vi "pH电极校准.vi"() -> ()   [LabVIEW 2016, in "斯坦道多参数.lvlib"]
uses:
  <vilib>/Utility/miscctls.llb/LVPointTypeDef.ctl
  <vilib>/Analysis/NI_AALBase.lvlib
  <vilib>/ptbypt/NI_PtbyPt.lvlib
panel:
  in  "刷新按钮":bool
  out "第三点信号值":dbl
  out "第二点信号值":dbl
  out "第一点信号值":dbl
  out "温度":dbl format="%#.2f"
  out "通讯状态":string
  out "电极状态标志":u16(ring) items=["OK", "第一点校正通过", "第二点校正通过", "校正失败,电极零点超出范围", "校正失败,电极斜率超出范围", "第三点校正通过"]
  in  "三点标液3":u16(ring)=6 caption="标液3" items=["TECH4.00", "TECH7.00", "TECH10.00", "NIST1.68", "NIST4.01", "NIST6.86", "NIST9.18", "NIST12.68"]
  in  "三点标液2":u16(ring)=5 caption="标液2" items=["TECH4.00", "TECH7.00", "TECH10.00", "NIST1.68", "NIST4.01", "NIST6.86", "NIST9.18", "NIST12.68"]
  in  "三点标液1":u16(ring)=4 caption="标液1" items=["TECH4.00", "TECH7.00", "TECH10.00", "NIST1.68", "NIST4.01", "NIST6.86", "NIST9.18", "NIST12.68"]
  out "第三点校准值":dbl
  in  "校准停止":bool
  in  "校准启动":bool
  out "第二点校准值":dbl
  out "第一点校准值":dbl
  out "提示":string
  in  "校准模式":enum16{"两点校准", "单点校准", "三点校准"}(ring)
  out "最小值":sgl format="%#.2f"
  out "最大值":sgl format="%#.2f"
  out "变异系数":dbl format="%#.6f"
  out "standard deviation":dbl caption="标准差" format="%#.2f"
  out "mean":dbl caption="均值" format="%#.2f"
  out "波形图表":dbl(graph) caption="历史曲线"
  out "当前检测值":dbl caption="测量值" format="%#.2f"
  out "标液2":dbl
  out "标液1":dbl
  out "当前信号值":dbl caption="信号值" format="%#.2f"
  out "偏移值补偿":dbl caption="pH偏移修正值" format="%#.2f"
  out "电极斜率":dbl format="%#.6f"
  out "电极零点":dbl format="%#.6f"
  # "酸碱度电极设定"
  # "℃"
  # "mV"
  # "mV"
  # "%"
  # "请选择校准模式:"
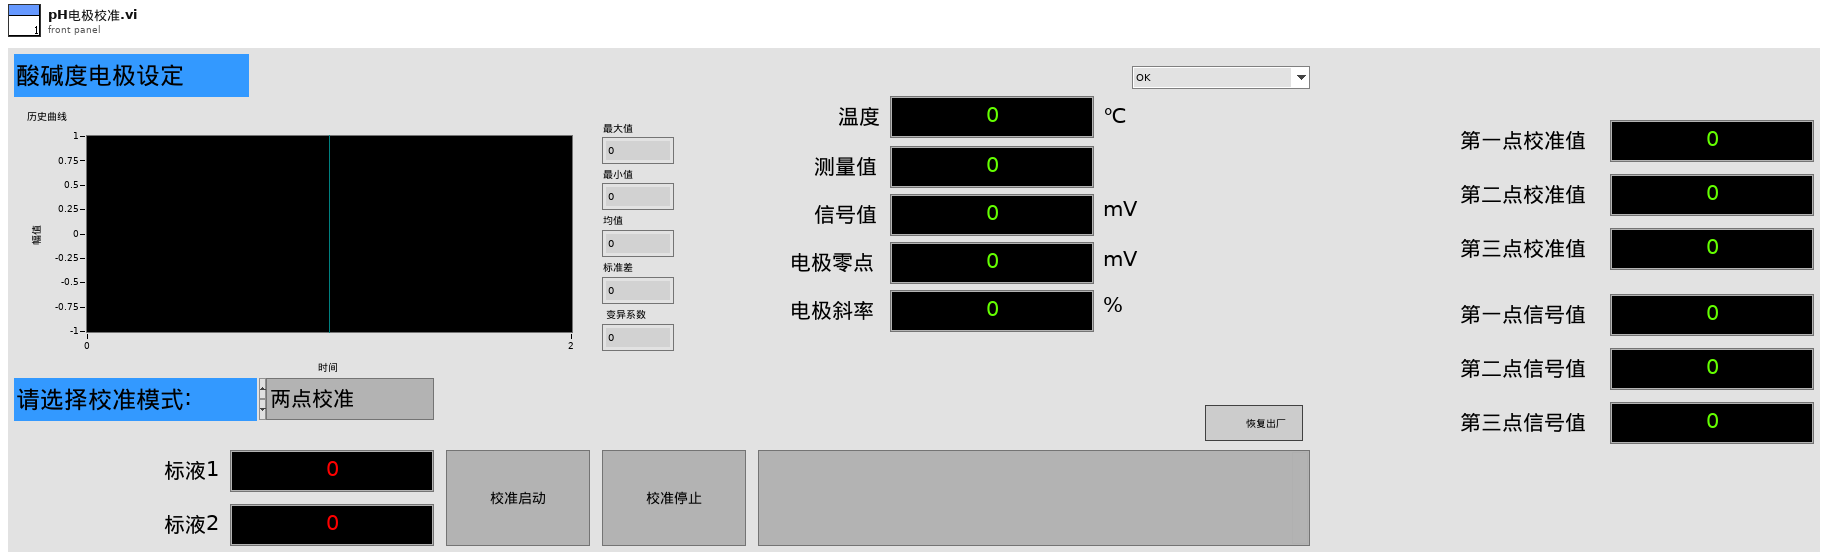
[diagram p1: front panel]
types:
  T1 = typedef "LVPointTypeDef.ctl" = cluster{"Horizontal":i16, "Vertical":i16}
  T2 = cluster{"电极状态标志":u16, "电极型号标志":u16, "酸碱度测量值":sgl, "温度测量值":sgl, "酸碱度信号值":sgl, "温度信号值":sgl, "酸碱度偏移修正值":sgl, "温度偏移修正值":sgl, "手动温度补偿值":sgl, "酸碱度电极零点":sgl, "酸碱度电极斜率":sgl, "第1点标准值记录":sgl, "第1点信号值记录":sgl, "第1点温度值记录":sgl, "第2点标准值记录":sgl, "第2点信号值记录":sgl, "第2点温度值记录":sgl, "命令滤波设定":u16, "温度模式":enum16{"ATC", "MTC"}, "生产批次":u16, "电极序号":u16, "串口地址":u16, "串口波特率":enum16{"9600", "19200", "115200"}, "串口校验位":enum16{"NONE", "ODD", "EVEN"}, "串口停止位":enum16{"1bit", "2bit"}, "第一点标准值":sgl, "第二点标准值":sgl}
  T3 = enum8{"Enabled", "Disabled", "Disabled and Grayed Out"}
  T4 = cluster{"ph":bool, "DO":bool, "Cond":bool, "Turb":bool, "叶绿素a":bool, "藻密度":bool, "ORP":bool}
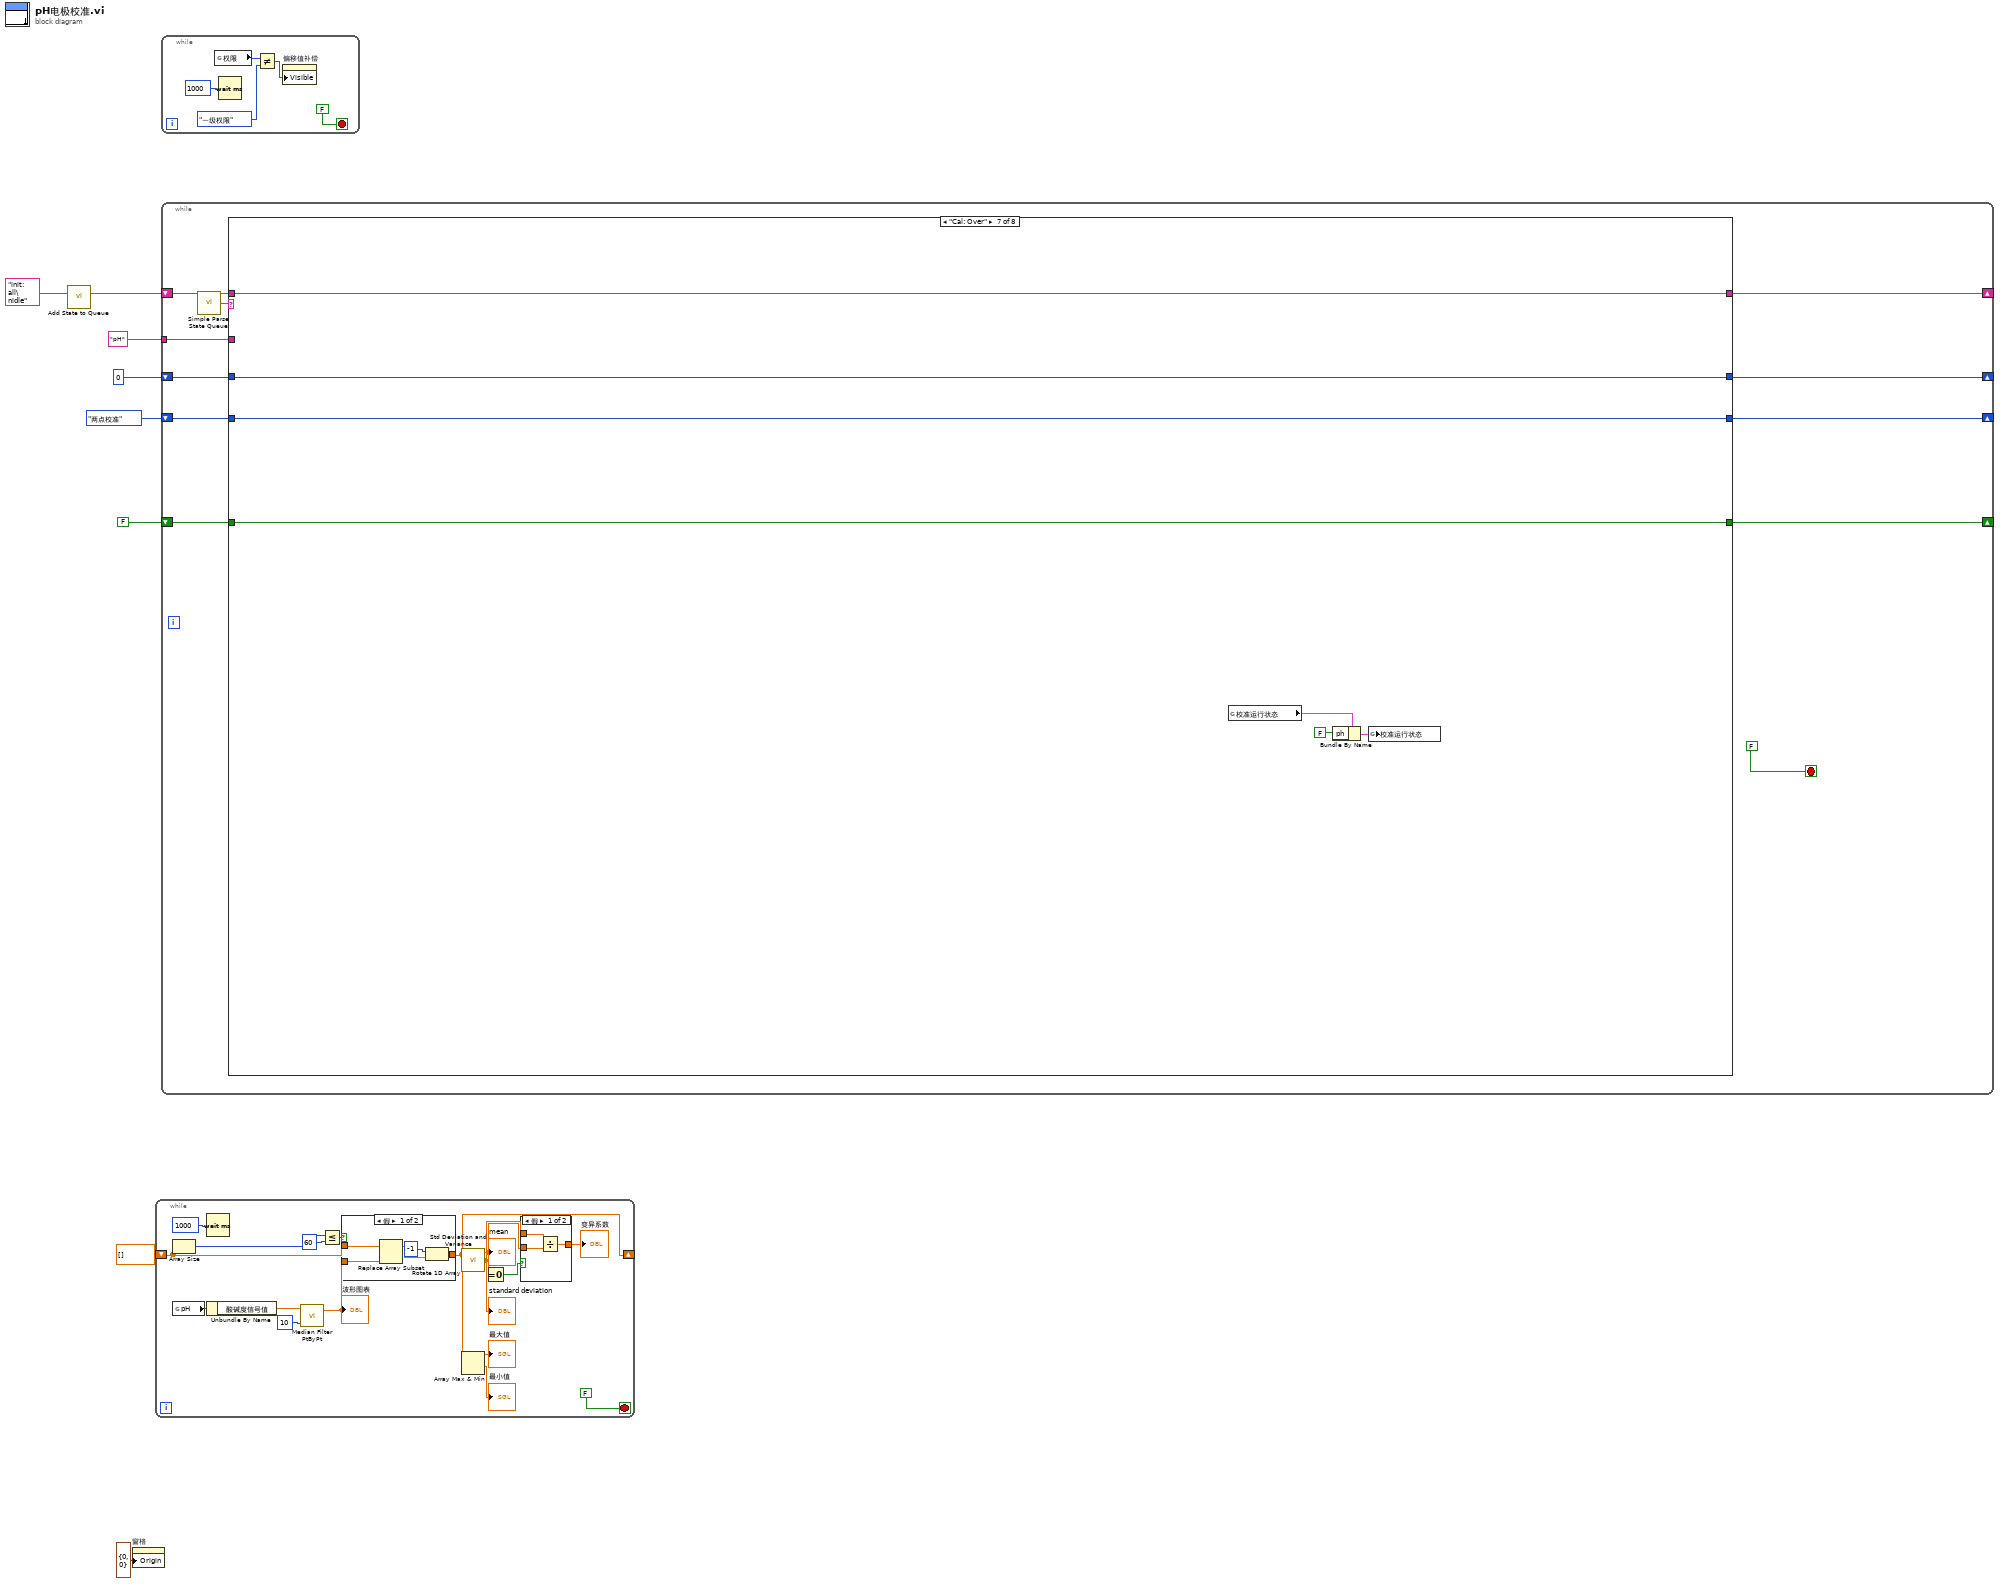
[diagram p0: block diagram]
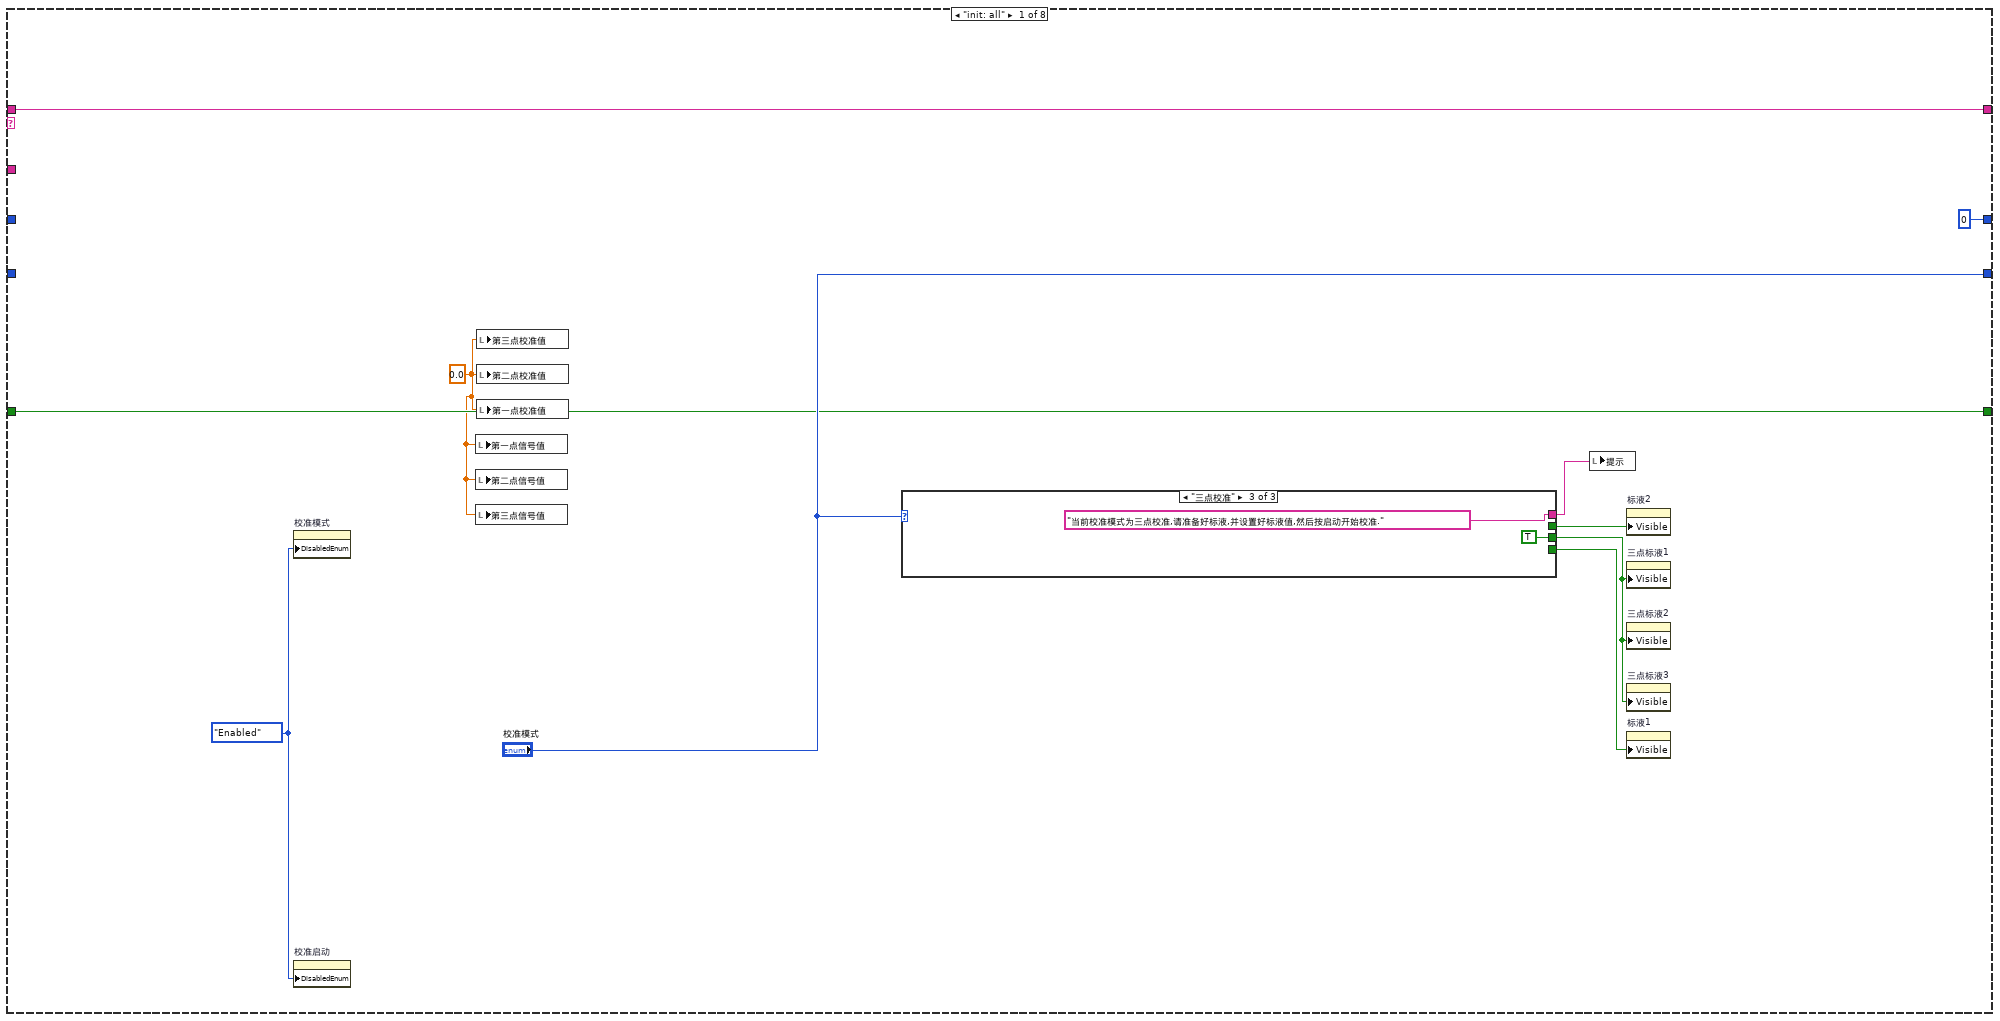
[diagram p2: hidden frame]
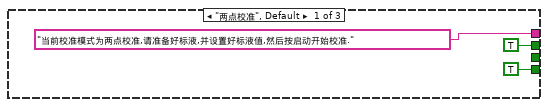
[diagram p3: hidden frame]
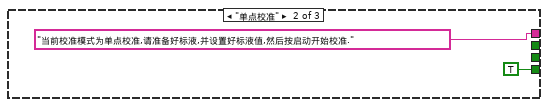
[diagram p4: hidden frame]
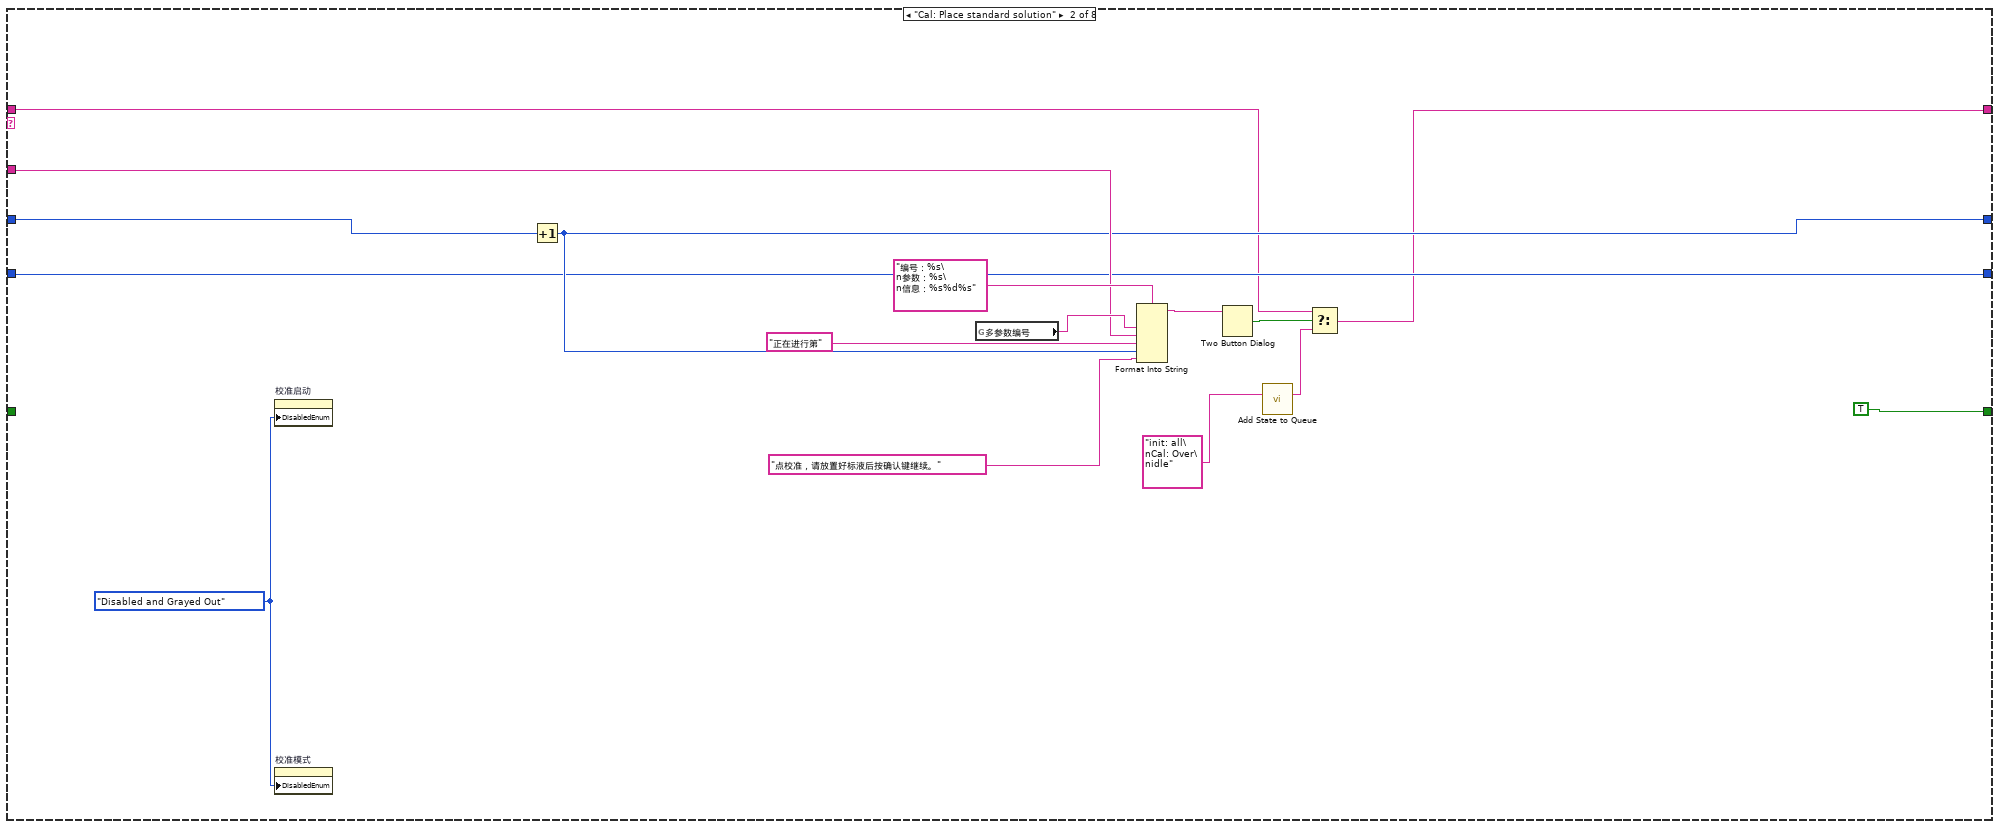
[diagram p5: hidden frame]
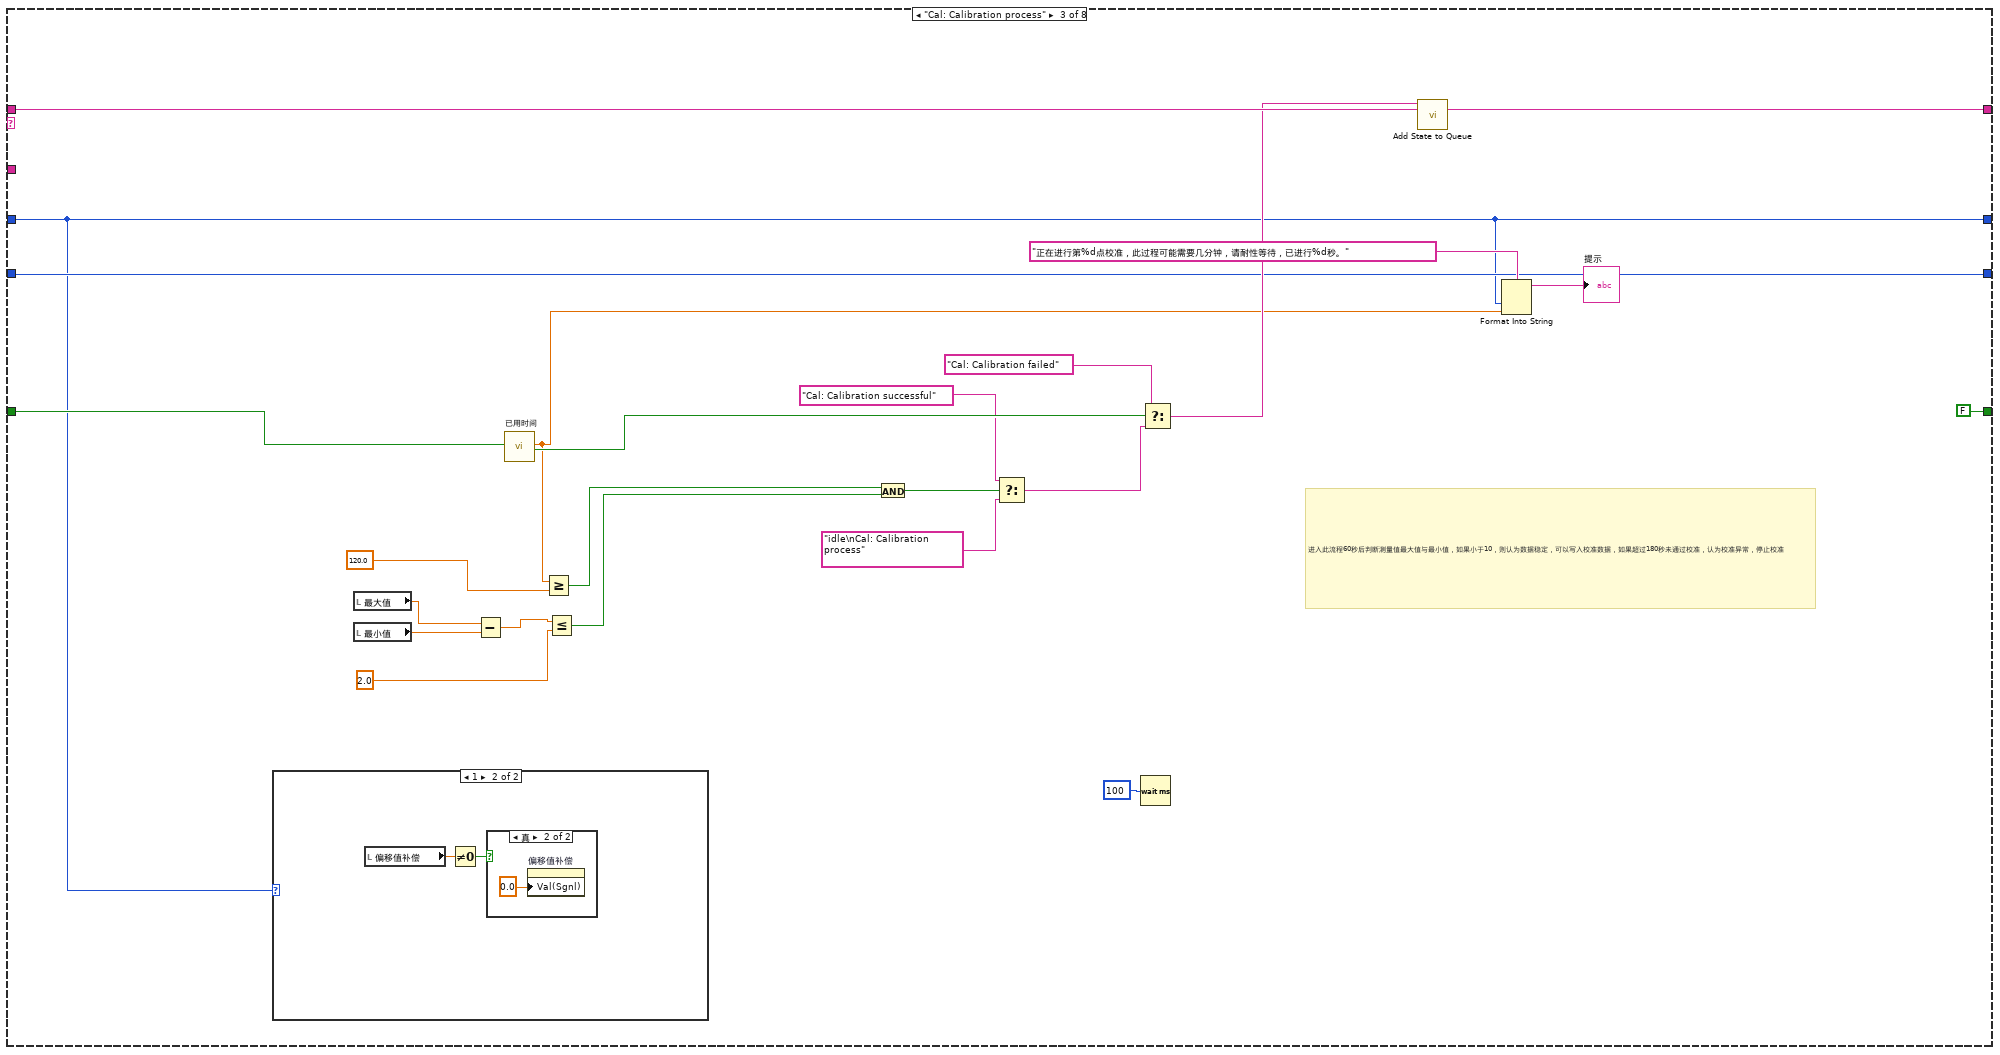
[diagram p6: hidden frame]
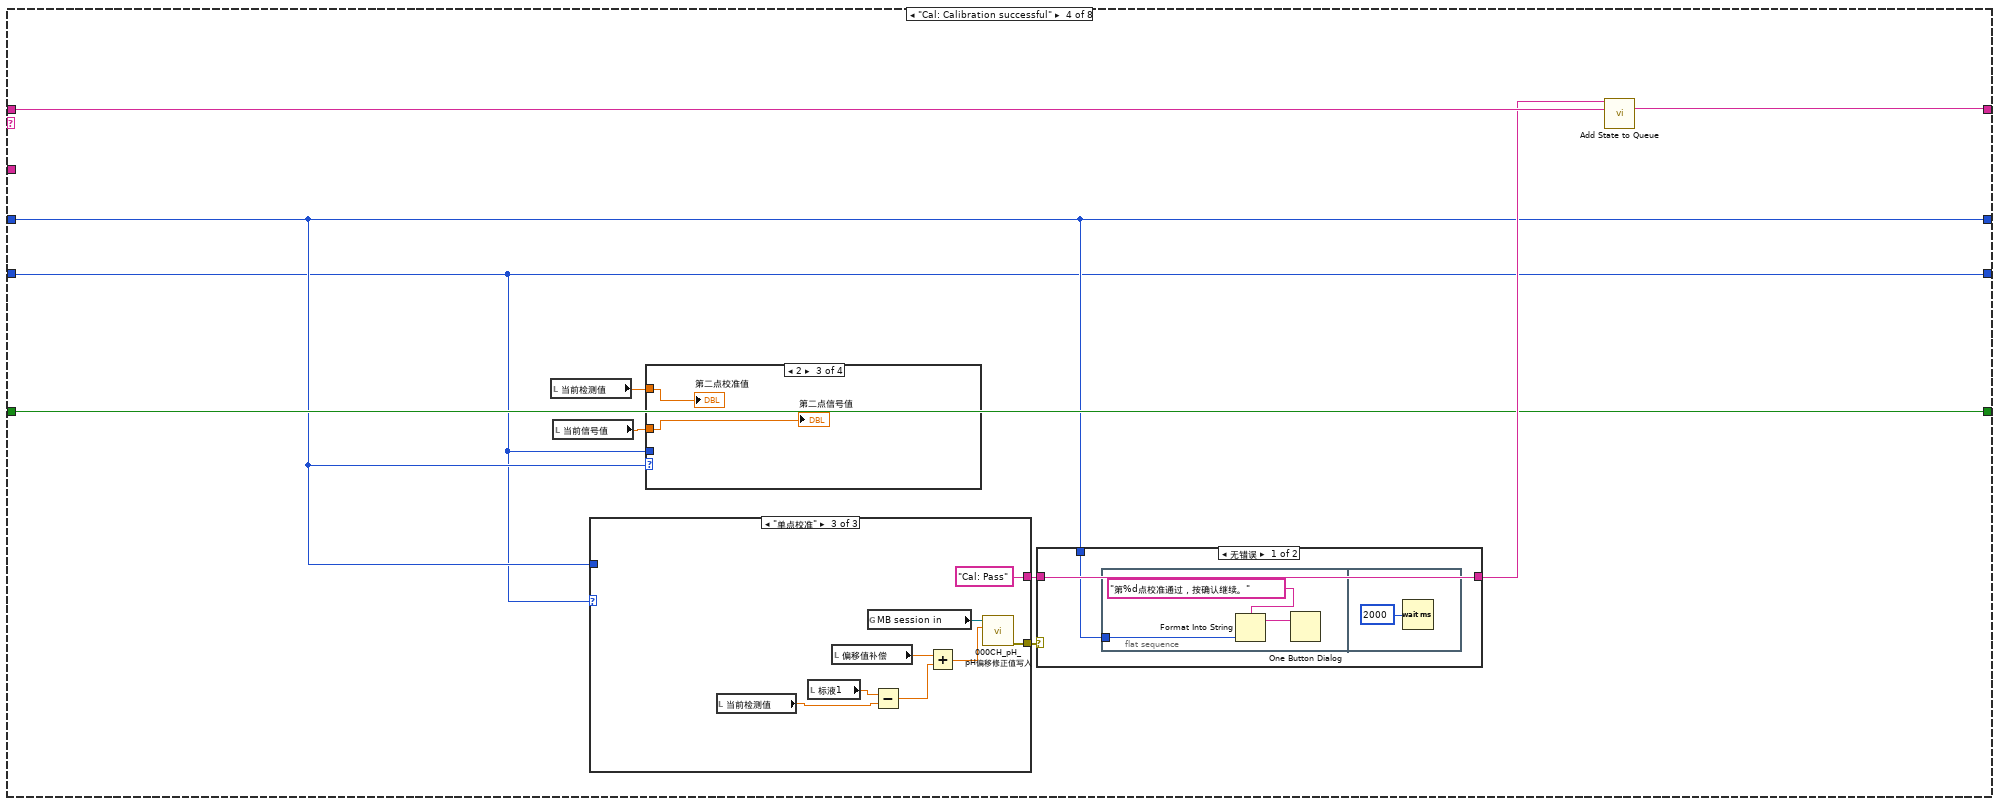
[diagram p9: hidden frame]
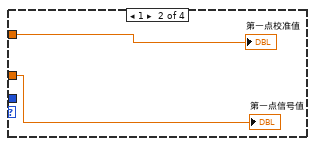
[diagram p11: hidden frame]
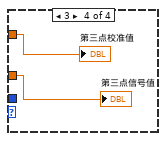
[diagram p12: hidden frame]
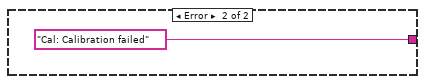
[diagram p13: hidden frame]
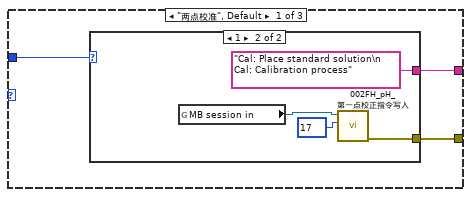
[diagram p14: hidden frame]
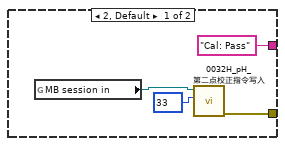
[diagram p15: hidden frame]
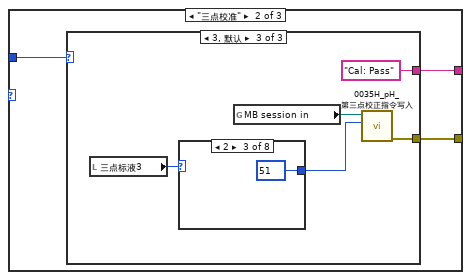
[diagram p16: hidden frame]
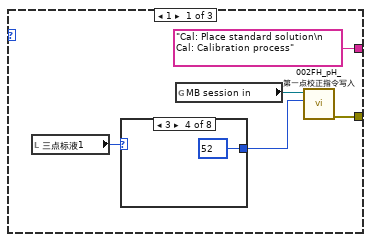
[diagram p17: hidden frame]
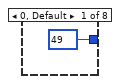
[diagram p18: hidden frame]
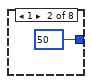
[diagram p19: hidden frame]
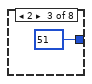
[diagram p20: hidden frame]
diagram:
  n1 = call "Add State to Queue.vi"("State(s) In (\"\")"="init: all\nidle" ("State(s) In (\"\")")) -> ("States Out"=w5:string)  [unwired: 14 in]
  n2 = property on="窗格" class="Pane"("Origin"=T1 {"Horizontal"=0, "Vertical"=0} ("原点")) -> ()  [unwired: 2 in, 2 out]
  n3 = while {
    shift-right: [w17] -> _
    shift-left: sgl[] [] -> [w21]
    stop <- FALSE stop-if-true
    n4 = Array Size(array=w21) -> (size(s)=w23:i32)
    n5 = global read "国弘过程全局变量.vi" "pH"() -> (w18:T2)
    n6 = Wait (ms)(milliseconds to wait=u32 1000 ("等待时间（毫秒）")) -> ()  [unwired: 1 out]
    n7 = Unbundle By Name(w18) -> ("酸碱度信号值"=w10:sgl)
    n8 = call <vilib>:"Median Filter PtByPt.vi"("rank"=10, "x"=w10) -> ("Filtered x"=w9:dbl)  [unwired: 2 in, 1 out]
    "波形图表" <- w9
    n9 = Less Or Equal?(x=w23, y=60) -> (x <= y?=w22:bool)
    n10 = case shown="假" w22 {
      tunnel: w21 -> [w33 w36]
      tunnel: w9 -> [w31 w35]
      tunnel: [w29 w34] -> w17
      frame False {
        n11 = Replace Array Subset(array=w33, new element=w31) -> (w32:sgl[])  [unwired: 1 in]
        n12 = Rotate 1D Array(1:w32, 2:-1 ("n")) -> (0:w29:sgl[])
      }
      frame True {
        n13 = Insert Into Array(array=w36, new element=w35) -> (w34:sgl[])  [unwired: 1 in]
      }
    }
    n14 = call <vilib>:"Std Deviation and Variance.vi"("X"=w17) -> ("mean"=w13:dbl, "standard deviation"=w12:dbl)  [unwired: 1 in, 1 out]
    "mean" <- w13
    "standard deviation" <- w12
    n15 = Array Max & Min(array=w17) -> (max value=→"最大值":sgl, min value=→"最小值":sgl)  [unwired: 2 out]
    n16 = Equal To 0?(x=w13) -> (x = 0?=w20:bool)
    n17 = case shown="假" w20 {
      tunnel: w12 -> [w28 _]
      tunnel: [w27 _] -> w14
      tunnel: w13 -> [w26 _]
      frame False {
        n18 = Divide(x=w28, y=w26) -> (x/y=w27:dbl)
      }
      frame True {
      }
    }
    "变异系数" <- w14
  }
  n19 = while {
    shift-right: [w44] -> _
    shift-left: w5 -> [w48]
    shift-right: [w41] -> _
    shift-left: 0 -> [w43]
    tunnel: "pH" ("State(s) In (\"\")") -> [w42]
    shift-right: [w39] -> _
    shift-left: enum16{"两点校准", "单点校准", "三点校准"}."两点校准" ("校准模式") -> [w40]
    shift-right: [w37] -> _
    shift-left: FALSE -> [w38]
    stop <- FALSE stop-if-true
    n20 = call "Simple Parse State Queue.vi"("State Queue"=w48) -> ("Remain States"=w45:string, "Next State"=w46:string)  [unwired: 13 in]
    n21 = case shown="\"Cal: Over\"" w46 {
      tunnel: w45 -> [w58 w68 w100 w116 _ _ w261 w271]
      tunnel: [w58 w67 w99 w115 w200 w207 w261 w270] -> w44
      tunnel: w43 -> [_ w77 w83 w110 w203 w216 w260 w268]
      tunnel: w42 -> [_ w78 _ _ w194 w212 _ _]
      tunnel: [0 w75 w83 w110 w203 w216 w260 w269] -> w41
      tunnel: w40 -> [_ w74 w84 w109 w202 w208 w259 w267]
      tunnel: ["校准模式" w74 w84 w109 w202 w208 w259 w267] -> w39
      tunnel: w38 -> [w51 _ w86 w111 w201 w211 w258 w265]
      tunnel: [w51 TRUE FALSE w111 w201 w211 w258 w265] -> w37
      frame "init: all" {
        w50 = T3."Enabled" ("禁用")
        w49 = 0.0 ("第一点校准值")
        n22 = property on="校准模式" class="Enum (严格)"("DisabledEnum"=w50) -> ()  [unwired: 2 in, 2 out]
        n23 = property on="校准启动" class="Bool"("DisabledEnum"=w50) -> ()  [unwired: 2 in, 2 out]
        n24 = local write "第一点信号值"(w49) -> ()
        n25 = local write "第二点信号值"(w49) -> ()
        n26 = local write "第三点信号值"(w49) -> ()
        n27 = local write "第三点校准值"(w49) -> ()
        n28 = local write "第二点校准值"(w49) -> ()
        n29 = local write "第一点校准值"(w49) -> ()
        n30 = case shown="\"三点校准\"" "校准模式" {
          tunnel: ["当前校准模式为两点校准,请准备好标液,并设置好标液值,然后按启动开始校准." ("提示") "当前校准模式为单点校准,请准备好标液,并设置好标液值,然后按启动开始校准." ("提示") "当前校准模式为三点校准,请准备好标液,并设置好标液值,然后按启动开始校准." ("提示")] -> w53
          tunnel: [TRUE ("可见") _ _] -> w57
          tunnel: [TRUE ("可见") TRUE ("可见") _] -> w55
          tunnel: [_ _ TRUE ("可见")] -> w56
          frame "两点校准", Default {
          }
          frame "单点校准" {
          }
          frame "三点校准" {
          }
        }
        n31 = local write "提示"(w53) -> ()
        n32 = property on="标液2" class="DigNum (严格)"("Visible"=w57) -> ()  [unwired: 2 in, 2 out]
        n33 = property on="三点标液1" class="Ring (严格)"("Visible"=w56) -> ()  [unwired: 2 in, 2 out]
        n34 = property on="三点标液2" class="Ring (严格)"("Visible"=w56) -> ()  [unwired: 2 in, 2 out]
        n35 = property on="三点标液3" class="Ring (严格)"("Visible"=w56) -> ()  [unwired: 2 in, 2 out]
        n36 = property on="标液1" class="DigNum (严格)"("Visible"=w55) -> ()  [unwired: 2 in, 2 out]
      }
      frame "Cal: Place standard solution" {
        w72 = T3."Disabled and Grayed Out" ("禁用")
        n37 = property on="校准启动" class="Bool"("DisabledEnum"=w72) -> ()  [unwired: 2 in, 2 out]
        n38 = property on="校准模式" class="Enum (严格)"("DisabledEnum"=w72) -> ()  [unwired: 2 in, 2 out]
        n39 = Increment(x=w77) -> (x+1=w75:i32)
        n40 = global read "多参数全局变量.vi" "多参数编号"() -> (w80:string)
        n41 = Format Into String(format string="编号：%s\n参数：%s\n信息：%s%d%s" ("格式字符串"), w80, w78, "正在进行第" ("消息"), w75, "点校准，请放置好标液后按确认键继续。" ("消息")) -> (resulting string=w71:string)  [unwired: 2 in, 1 out]
        n42 = Two Button Dialog(message=w71) -> (T button?=w70:bool)  [unwired: 2 in]
        n43 = call "Add State to Queue.vi"("State(s) In (\"\")"="init: all\nCal: Over\nidle" ("State(s) In (\"\")")) -> ("States Out"=w69:string)  [unwired: 14 in]
        n44 = Select(t=w68, s=w70, f=w69) -> (s? t:f=w67:string)
      }
      frame "Cal: Calibration process" {
        # "进入此流程60秒后判断测量值最大值与最小值，如果小于10，则认为数据稳定，可以写入校准数据，如果超过180秒未通过校准，认为校准异常，停止校准"
        n45 = case shown="1" w83 {
          frame 0, Default {
          }
          frame 1 {
            n46 = local read "偏移值补偿"() -> (w106:dbl)
            n47 = Not Equal To 0?(x=w106) -> (x != 0?=w107:bool)
            n48 = case shown="真" w107 {
              frame False {
              }
              frame True {
                n49 = property on="偏移值补偿" class="DigNum (严格)"("Val(Sgnl)"=0.0 ("值(信号)")) -> ()  [unwired: 2 in, 2 out]
              }
            }
          }
        }
        n50 = local read "最大值"() -> (w104:sgl)
        n51 = local read "最小值"() -> (w103:sgl)
        n52 = Subtract(x=w104, y=w103) -> (x-y=w105:sgl)
        n53 = call "已用时间"("Reset"=w86) -> ("Elapsed Time (s)"=w82:dbl, "Time has Elapsed"=w101:bool)  [unwired: 11 in, 6 out]
        n54 = Greater Or Equal?(x=w82, y=120.0) -> (x >= y?=w96:bool)
        n55 = Less Or Equal?(x=w105, y=2.0) -> (x <= y?=w92:bool)
        n56 = And(x=w96, y=w92) -> (x .and. y?=w93:bool)
        n57 = Select(t="Cal: Calibration successful" ("State(s) In (\"\")"), s=w93, f="idle\nCal: Calibration process" ("State(s) In (\"\")")) -> (s? t:f=w91:string)
        n58 = Wait (ms)(milliseconds to wait=u32 100 ("等待时间（毫秒）")) -> ()  [unwired: 1 out]
        n59 = Select(t="Cal: Calibration failed" ("State(s) In (\"\")"), s=w101, f=w91) -> (s? t:f=w90:string)
        n60 = call "Add State to Queue.vi"("State(s) In Front (\"\")"=w90, "State(s) In (\"\")"=w100) -> ("States Out"=w99:string)  [unwired: 13 in]
        n61 = Format Into String(format string="正在进行第%d点校准，此过程可能需要几分钟，请耐性等待，已进行%d秒。" ("格式字符串"), w83, w82) -> (resulting string=→"提示":string)  [unwired: 2 in, 1 out]
      }
      frame "Cal: Calibration successful" {
        n62 = local read "当前检测值"() -> (w112:dbl)
        n63 = local read "当前信号值"() -> (w113:dbl)
        n64 = case shown="\"单点校准\"" w109 {
          tunnel: [w134 w145 w187] -> w118
          tunnel: [w133 w143 "Cal: Pass" ("State(s) In (\"\")")] -> w117
          tunnel: w110 -> [w132 w144 _]
          frame "两点校准", Default {
            n65 = case shown="1" w132 {
              tunnel: [w135 w140] -> w134
              tunnel: ["Cal: Pass" ("State(s) In (\"\")") "Cal: Place standard solution\n Cal: Calibration process" ("State(s) In (\"\")")] -> w133
              frame 2, Default {
                n66 = global read "多参数全局变量.vi" "MB session in"() -> (w137:refnum<class "MB_Master.lvclass">)
                n67 = call "0032H_pH_第二点校正指令写入.vi"("数值"=u16 33, "MB session in"=w137) -> ("error out"=w135:errorcluster)  [unwired: 8 in, 1 out]
              }
              frame 1 {
                n68 = global read "多参数全局变量.vi" "MB session in"() -> (w142:refnum<class "MB_Master.lvclass">)
                n69 = call "002FH_pH_第一点校正指令写入.vi"("数值"=u16 17, "MB session in"=w142) -> ("error out"=w140:errorcluster)  [unwired: 8 in, 1 out]
              }
            }
          }
          frame "三点校准" {
            n70 = case shown="3, 默认" w144 {
              tunnel: [w147 w160 w173] -> w145
              tunnel: ["Cal: Place standard solution\n Cal: Calibration process" ("State(s) In (\"\")") "Cal: Place standard solution\n Cal: Calibration process" ("State(s) In (\"\")") "Cal: Pass" ("State(s) In (\"\")")] -> w143
              frame 1 {
                n71 = local read "三点标液1"() -> (w149:u16)
                n72 = case shown="3" w149 {
                  tunnel: [u16 49 ("数值") u16 50 ("数值") u16 51 ("数值") u16 52 ("数值") u16 53 ("数值") u16 54 ("数值") u16 55 ("数值") u16 56 ("数值")] -> w148
                  frame 0, Default {
                  }
                  frame 1 {
                  }
                  frame 2 {
                  }
                  frame 3 {
                  }
                  frame 4 {
                  }
                  frame 5 {
                  }
                  frame 6 {
                  }
                  frame 7 {
                  }
                }
                n73 = global read "多参数全局变量.vi" "MB session in"() -> (w150:refnum<class "MB_Master.lvclass">)
                n74 = call "002FH_pH_第一点校正指令写入.vi"("数值"=w148, "MB session in"=w150) -> ("error out"=w147:errorcluster)  [unwired: 8 in, 1 out]
              }
              frame 2 {
                n75 = local read "三点标液2"() -> (w162:u16)
                n76 = case shown="7" w162 {
                  tunnel: [u16 49 ("数值") u16 50 ("数值") u16 51 ("数值") u16 52 ("数值") u16 53 ("数值") u16 54 ("数值") u16 55 ("数值") u16 56 ("数值")] -> w161
                  frame 0, Default {
                  }
                  frame 1 {
                  }
                  frame 2 {
                  }
                  frame 3 {
                  }
                  frame 4 {
                  }
                  frame 5 {
                  }
                  frame 6 {
                  }
                  frame 7 {
                  }
                }
                n77 = global read "多参数全局变量.vi" "MB session in"() -> (w163:refnum<class "MB_Master.lvclass">)
                n78 = call "0032H_pH_第二点校正指令写入.vi"("数值"=w161, "MB session in"=w163) -> ("error out"=w160:errorcluster)  [unwired: 8 in, 1 out]
              }
              frame 3, Default {
                n79 = local read "三点标液3"() -> (w175:u16)
                n80 = case shown="2" w175 {
                  tunnel: [u16 49 ("数值") u16 50 ("数值") u16 51 ("数值") u16 52 ("数值") u16 53 ("数值") u16 54 ("数值") u16 55 ("数值") u16 56 ("数值")] -> w174
                  frame 0, Default {
                  }
                  frame 1 {
                  }
                  frame 2 {
                  }
                  frame 3 {
                  }
                  frame 4 {
                  }
                  frame 5 {
                  }
                  frame 6 {
                  }
                  frame 7 {
                  }
                }
                n81 = global read "多参数全局变量.vi" "MB session in"() -> (w176:refnum<class "MB_Master.lvclass">)
                n82 = call "0035H_pH_第三点校正指令写入.vi"("数值"=w174, "MB session in"=w176) -> ("error out"=w173:errorcluster)  [unwired: 8 in, 1 out]
              }
            }
          }
          frame "单点校准" {
            n83 = local read "当前检测值"() -> (w185:dbl)
            n84 = local read "标液1"() -> (w192:dbl)
            n85 = local read "偏移值补偿"() -> (w188:dbl)
            n86 = global read "多参数全局变量.vi" "MB session in"() -> (w191:refnum<class "MB_Master.lvclass">)
            n87 = Subtract(x=w192, y=w185) -> (x-y=w190:dbl)
            n88 = Add(x=w188, y=w190) -> (x+y=w189:dbl)
            n89 = call "000CH_pH_pH偏移修正值写入.vi"("数值"=w189, "MB session in"=w191) -> ("error out"=w187:errorcluster)  [unwired: 8 in, 1 out]
          }
        }
        n90 = case shown="2" w110 {
          tunnel: w113 -> [_ w120 w121 w123]
          tunnel: w112 -> [_ w119 w122 w124]
          tunnel: w109 -> [_ _ _ _]
          frame 0, Default {
          }
          frame 1 {
            "第一点校准值" <- w119
            "第一点信号值" <- w120
          }
          frame 2 {
            "第二点校准值" <- w122
            "第二点信号值" <- w121
          }
          frame 3 {
            "第三点校准值" <- w124
            "第三点信号值" <- w123
          }
        }
        n91 = case shown="无错误" w118 {
          tunnel: w117 -> [w126 _]
          tunnel: [w126 "Cal: Calibration failed" ("State(s) In (\"\")")] -> w114
          tunnel: w110 -> [w125 _]
          frame No Error {
            n92 = flat-sequence {
              tunnel: w125 -> [w127]
              frame #0 {
                n93 = Format Into String(format string="第%d点校准通过，按确认继续。" ("格式字符串"), w127) -> (resulting string=w129:string)  [unwired: 2 in, 1 out]
                n94 = One Button Dialog(message=w129) -> ()  [unwired: 1 in, 1 out]
              }
              frame #1 {
                n95 = Wait (ms)(milliseconds to wait=u32 2000 ("等待时间（毫秒）")) -> ()  [unwired: 1 out]
              }
            }
          }
          frame Error {
          }
        }
        n96 = call "Add State to Queue.vi"("State(s) In Front (\"\")"=w114, "State(s) In (\"\")"=w116) -> ("States Out"=w115:string)  [unwired: 13 in]
      }
      frame "Cal: Calibration failed" {
        n97 = global read "多参数全局变量.vi" "多参数编号"() -> (w197:string)
        n98 = call "Add State to Queue.vi"("State(s) In (\"\")"="init: all\nCal: Over\nidle" ("State(s) In (\"\")")) -> ("States Out"=w200:string)  [unwired: 14 in]
        n99 = Format Into String(format string="编号：%s\n参数：%s\n信息：%s" ("格式字符串"), w197, w194, "校准失败！" ("消息")) -> (resulting string=w196:string)  [unwired: 2 in, 1 out]
        n100 = One Button Dialog(message=w196) -> ()  [unwired: 1 in, 1 out]
        n101 = call "校准日志.vi"("table"="校准记录", "日志信息"=w196) -> ()  [unwired: 9 in, 1 out]
      }
      frame "Cal: Pass" {
        n102 = flat-sequence {
          tunnel: [w221] -> w209
          tunnel: w208 -> [w220]
          tunnel: [w219] -> w206
          tunnel: [w218] -> w205
          frame #0 {
            n103 = Wait (ms)(milliseconds to wait=u32 3000 ("等待时间（毫秒）")) -> ()  [unwired: 1 out]
          }
          frame #1 {
            n104 = global read "国弘过程全局变量.vi" "pH"() -> (w222:T2)
            n105 = Unbundle By Name(w222) -> ("电极状态标志"=w223:u16, "酸碱度电极零点"=w219:sgl, "酸碱度电极斜率"=w218:sgl)
            n106 = case shown="\"两点校准\", 默认" w220 {
              tunnel: [w225 w240 w257] -> w221
              tunnel: w223 -> [w224 w239 _]
              frame "两点校准", Default {
                n107 = case shown="2" w224 {
                  selector: w224 -> [_ _ w236]
                  tunnel: ["校准异常，校准未完成。" ("格式字符串") w234 w235] -> w225
                  frame 0, Default {
                  }
                  frame 2 {
                    n108 = local read "第一点校准值"() -> (w232:dbl)
                    n109 = local read "第一点信号值"() -> (w233:dbl)
                    n110 = local read "第二点校准值"() -> (w229:dbl)
                    n111 = local read "第二点信号值"() -> (w228:dbl)
                    n112 = local read "标液1"() -> (w230:dbl)
                    n113 = local read "标液2"() -> (w227:dbl)
                    n114 = Format Into String(format string="校准结果：\n第一点校准值=%#.2f，第一点信号值=%#.2f mV，第一点标准值=%#.2f；\n第二点校准值=%#.2f，第二点信号值=%#.2f mV，第二点标准值=%#.2f。" ("提示"), w232, w233, w230, w229, w228, w227) -> (resulting string=w234:string)  [unwired: 2 in, 1 out]
                  }
                  frame 3, 4 {
                    n115 = case shown="4" w236 {
                      tunnel: ["校正失败，电极零点超出范围" "校正失败，电极斜率超出范围"] -> w235
                      frame 3, Default {
                      }
                      frame 4 {
                      }
                    }
                  }
                }
              }
              frame "三点校准" {
                n116 = case shown="5" w239 {
                  tunnel: ["校准异常，校准未完成。" ("格式字符串") w252] -> w240
                  frame 0, Default {
                  }
                  frame 5 {
                    n117 = local read "第一点校准值"() -> (w251:dbl)
                    n118 = local read "第一点信号值"() -> (w249:dbl)
                    n119 = local read "第二点校准值"() -> (w247:dbl)
                    n120 = local read "第二点信号值"() -> (w246:dbl)
                    n121 = local read "第三点校准值"() -> (w244:dbl)
                    n122 = local read "第三点信号值"() -> (w243:dbl)
                    n123 = property on="三点标液1" class="Ring (严格)"() -> ("RingText.Text"=w248:string)  [unwired: 2 in, 2 out]
                    n124 = property on="三点标液2" class="Ring (严格)"() -> ("RingText.Text"=w245:string)  [unwired: 2 in, 2 out]
                    n125 = property on="三点标液3" class="Ring (严格)"() -> ("RingText.Text"=w242:string)  [unwired: 2 in, 2 out]
                    n126 = Format Into String(format string="校准结果：\n第一点校准值=%#.2f，第一点信号值=%#.2f mV，第一点标准值=%s；\n第二点校准值=%#.2f，第二点信号值=%#.2f mV，第二点标准值=%s；\n第三点校准值=%#.2f，第三点信号值=%#.2f mV，第三点标准值=%s。" ("提示"), w251, w249, w248, w247, w246, w245, w244, w243, w242) -> (resulting string=w252:string)  [unwired: 2 in, 1 out]
                  }
                }
              }
              frame "单点校准" {
                n127 = local read "第一点校准值"() -> (w256:dbl)
                n128 = local read "第一点信号值"() -> (w254:dbl)
                n129 = local read "标液1"() -> (w253:dbl)
                n130 = Format Into String(format string="校准结果：\n校准值=%#.2f，信号值=%#.2f，标准值=%#.2f。" ("提示"), w256, w254, w253) -> (resulting string=w257:string)  [unwired: 2 in, 1 out]
              }
            }
          }
        }
        n131 = call "Add State to Queue.vi"("State(s) In (\"\")"="init: all\nCal: Over\nidle" ("State(s) In (\"\")")) -> ("States Out"=w207:string)  [unwired: 14 in]
        n132 = global read "多参数全局变量.vi" "多参数编号"() -> (w213:string)
        n133 = Format Into String(format string="编号：%s\n参数：%s\n信息：%s\n电极零点=%#.2f，电极斜率=%#.2f%%。" ("格式字符串"), w213, w212, w209, w206, w205) -> (resulting string=w210:string)  [unwired: 2 in, 1 out]
        n134 = One Button Dialog(message=w210) -> ()  [unwired: 1 in, 1 out]
        n135 = call "校准日志.vi"("table"="校准记录", "日志信息"=w210) -> ()  [unwired: 9 in, 1 out]
      }
      frame "Cal: Over" {
        n136 = global read "多参数全局变量.vi" "校准运行状态"() -> (w263:T4)
        n137 = Bundle By Name(cluster=w263, "ph"=FALSE) -> (w264:T4)
        n138 = global write "多参数全局变量.vi" "校准运行状态"(w264) -> ()
      }
      frame "idle", Default {
        n139 = event shown="[10] \"校准启动\": 值改变" {
          selector: _ -> [_ _ _ _ _ _ _ _ _ _ _ _]
          dyn-events: _ -> [_ _ _ _ _ _ _ _ _ _ _ _]
          timeout: 10 -> [_ _ _ _ _ _ _ _ _ _ _ _]
          tunnel: [_ _ _ _ _ _ w356 w366 w372 _ _ _] -> _
          tunnel: w271 -> [w288 w292 w293 w315 w329 w347 w361 w362 w368 w376 w387 _]
          tunnel: [w287 w291 w294 w316 w330 w348 w360 w363 w369 w375 w386 w389] -> w270
          tunnel: [w286 w289 w295 w317 w331 w350 w359 w364 w370 w374 w384 w390] -> w269
          tunnel: w268 -> [w286 w289 w295 w317 w331 w350 w359 w364 w370 w374 w384 w390]
          event Timeout {
            n140 = event-data() -> ()  [unwired: 1 in, 3 out]
            n141 = global read "国弘过程全局变量.vi" "pH"() -> (w285:T2)
            n142 = Unbundle By Name(w285) -> ("电极状态标志"=→"电极状态标志":u16, "酸碱度电极零点"=→"电极零点":sgl, "酸碱度电极斜率"=→"电极斜率":sgl, "酸碱度偏移修正值"=→"偏移值补偿":sgl, "酸碱度信号值"=→"当前信号值":sgl, "第一点标准值"=→"标液1":sgl, "第二点标准值"=→"标液2":sgl, "酸碱度测量值"=→"当前检测值":sgl, "温度测量值"=→"温度":sgl)  [unwired: 1 out]
            n143 = global read "多参数全局变量.vi" "ph通讯状态"() -> (w274:bool)
            n144 = property on="通讯状态" class="Str"("Blinking"=TRUE ("闪烁"), "Text.BG Color"=u32 16711680, "Visible"=w274) -> ()  [unwired: 2 in, 2 out]
            n145 = call "Add State to Queue.vi"("State(s) In (\"\")"=w288) -> ("States Out"=w287:string)  [unwired: 14 in]
            "通讯状态" <- "通讯异常" ("当前串口")
          }
          event "校准模式": Value Change {
            n146 = event-data() -> ()  [unwired: 1 in, 6 out]
            n147 = call "Add State to Queue.vi"("State(s) In (\"\")"=w292, "State(s) At Back (\"\")"="init: all\nidle" ("State(s) In (\"\")")) -> ("States Out"=w291:string)  [unwired: 13 in]
          }
          event "三点标液1": Value Change {
            n148 = event-data() -> ("NewVal"=w296:u16)  [unwired: 1 in, 5 out]
            n149 = case shown="1" w296 {
              frame 0, Default {
                w297 = u16 0 items=["TECH4.00", "TECH7.00", "TECH10.00", "NIST1.68", "NIST4.01", "NIST6.86", "NIST9.18", "NIST12.68"] ("标液2")
                w298 = u16 2 items=["TECH4.00", "TECH7.00", "TECH10.00", "NIST1.68", "NIST4.01", "NIST6.86", "NIST9.18", "NIST12.68"] ("标液3")
                w299 = u16 1 items=["TECH4.00", "TECH7.00", "TECH10.00", "NIST1.68", "NIST4.01", "NIST6.86", "NIST9.18", "NIST12.68"] ("标液2")
                n150 = local write "三点标液3"(w298) -> ()
                n151 = local write "三点标液2"(w299) -> ()
                n152 = local write "三点标液1"(w297) -> ()
              }
              frame 1 {
                w300 = u16 0 items=["TECH4.00", "TECH7.00", "TECH10.00", "NIST1.68", "NIST4.01", "NIST6.86", "NIST9.18", "NIST12.68"] ("标液2")
                w301 = u16 2 items=["TECH4.00", "TECH7.00", "TECH10.00", "NIST1.68", "NIST4.01", "NIST6.86", "NIST9.18", "NIST12.68"] ("标液3")
                w302 = u16 1 items=["TECH4.00", "TECH7.00", "TECH10.00", "NIST1.68", "NIST4.01", "NIST6.86", "NIST9.18", "NIST12.68"] ("标液2")
                n153 = local write "三点标液3"(w301) -> ()
                n154 = local write "三点标液2"(w302) -> ()
                n155 = local write "三点标液1"(w300) -> ()
              }
              frame 2 {
                w303 = u16 2 items=["TECH4.00", "TECH7.00", "TECH10.00", "NIST1.68", "NIST4.01", "NIST6.86", "NIST9.18", "NIST12.68"] ("标液2")
                w304 = u16 0 items=["TECH4.00", "TECH7.00", "TECH10.00", "NIST1.68", "NIST4.01", "NIST6.86", "NIST9.18", "NIST12.68"] ("标液3")
                w305 = u16 1 items=["TECH4.00", "TECH7.00", "TECH10.00", "NIST1.68", "NIST4.01", "NIST6.86", "NIST9.18", "NIST12.68"] ("标液2")
                n156 = local write "三点标液3"(w304) -> ()
                n157 = local write "三点标液2"(w305) -> ()
                n158 = local write "三点标液1"(w303) -> ()
              }
              frame 3 {
                w306 = u16 3 items=["TECH4.00", "TECH7.00", "TECH10.00", "NIST1.68", "NIST4.01", "NIST6.86", "NIST9.18", "NIST12.68"] ("标液2")
                w307 = u16 5 items=["TECH4.00", "TECH7.00", "TECH10.00", "NIST1.68", "NIST4.01", "NIST6.86", "NIST9.18", "NIST12.68"] ("标液3")
                w308 = u16 4 items=["TECH4.00", "TECH7.00", "TECH10.00", "NIST1.68", "NIST4.01", "NIST6.86", "NIST9.18", "NIST12.68"] ("标液2")
                n159 = local write "三点标液3"(w307) -> ()
                n160 = local write "三点标液2"(w308) -> ()
                n161 = local write "三点标液1"(w306) -> ()
              }
              frame 4 {
                w309 = u16 4 items=["TECH4.00", "TECH7.00", "TECH10.00", "NIST1.68", "NIST4.01", "NIST6.86", "NIST9.18", "NIST12.68"] ("标液2")
                w310 = u16 6 items=["TECH4.00", "TECH7.00", "TECH10.00", "NIST1.68", "NIST4.01", "NIST6.86", "NIST9.18", "NIST12.68"] ("标液3")
                w311 = u16 5 items=["TECH4.00", "TECH7.00", "TECH10.00", "NIST1.68", "NIST4.01", "NIST6.86", "NIST9.18", "NIST12.68"] ("标液2")
                n162 = local write "三点标液3"(w310) -> ()
                n163 = local write "三点标液2"(w311) -> ()
                n164 = local write "三点标液1"(w309) -> ()
              }
              frame 5..7 {
                w312 = u16 5 items=["TECH4.00", "TECH7.00", "TECH10.00", "NIST1.68", "NIST4.01", "NIST6.86", "NIST9.18", "NIST12.68"] ("标液2")
                w313 = u16 7 items=["TECH4.00", "TECH7.00", "TECH10.00", "NIST1.68", "NIST4.01", "NIST6.86", "NIST9.18", "NIST12.68"] ("标液3")
                w314 = u16 6 items=["TECH4.00", "TECH7.00", "TECH10.00", "NIST1.68", "NIST4.01", "NIST6.86", "NIST9.18", "NIST12.68"] ("标液2")
                n165 = local write "三点标液3"(w313) -> ()
                n166 = local write "三点标液2"(w314) -> ()
                n167 = local write "三点标液1"(w312) -> ()
              }
            }
            n168 = call "Add State to Queue.vi"("State(s) In (\"\")"=w293) -> ("States Out"=w294:string)  [unwired: 14 in]
          }
          event "三点标液2": Value Change {
            n169 = event-data() -> ("NewVal"=w318:u16)  [unwired: 1 in, 5 out]
            n170 = case shown="6, 7" w318 {
              frame 0..2, Default {
                w319 = u16 0 items=["TECH4.00", "TECH7.00", "TECH10.00", "NIST1.68", "NIST4.01", "NIST6.86", "NIST9.18", "NIST12.68"] ("标液2")
                w320 = u16 2 items=["TECH4.00", "TECH7.00", "TECH10.00", "NIST1.68", "NIST4.01", "NIST6.86", "NIST9.18", "NIST12.68"] ("标液3")
                w321 = u16 1 items=["TECH4.00", "TECH7.00", "TECH10.00", "NIST1.68", "NIST4.01", "NIST6.86", "NIST9.18", "NIST12.68"] ("标液2")
                n171 = local write "三点标液3"(w320) -> ()
                n172 = local write "三点标液2"(w321) -> ()
                n173 = local write "三点标液1"(w319) -> ()
              }
              frame 3, 4 {
                w322 = u16 3 items=["TECH4.00", "TECH7.00", "TECH10.00", "NIST1.68", "NIST4.01", "NIST6.86", "NIST9.18", "NIST12.68"] ("标液2")
                w323 = u16 5 items=["TECH4.00", "TECH7.00", "TECH10.00", "NIST1.68", "NIST4.01", "NIST6.86", "NIST9.18", "NIST12.68"] ("标液3")
                w324 = u16 4 items=["TECH4.00", "TECH7.00", "TECH10.00", "NIST1.68", "NIST4.01", "NIST6.86", "NIST9.18", "NIST12.68"] ("标液2")
                n174 = local write "三点标液3"(w323) -> ()
                n175 = local write "三点标液2"(w324) -> ()
                n176 = local write "三点标液1"(w322) -> ()
              }
              frame 5 {
                w325 = u16 6 items=["TECH4.00", "TECH7.00", "TECH10.00", "NIST1.68", "NIST4.01", "NIST6.86", "NIST9.18", "NIST12.68"] ("标液3")
                w326 = u16 5 items=["TECH4.00", "TECH7.00", "TECH10.00", "NIST1.68", "NIST4.01", "NIST6.86", "NIST9.18", "NIST12.68"] ("标液2")
                n177 = local write "三点标液3"(w325) -> ()
                n178 = local write "三点标液2"(w326) -> ()
              }
              frame 6, 7 {
                w327 = u16 7 items=["TECH4.00", "TECH7.00", "TECH10.00", "NIST1.68", "NIST4.01", "NIST6.86", "NIST9.18", "NIST12.68"] ("标液3")
                w328 = u16 6 items=["TECH4.00", "TECH7.00", "TECH10.00", "NIST1.68", "NIST4.01", "NIST6.86", "NIST9.18", "NIST12.68"] ("标液2")
                n179 = local write "三点标液3"(w327) -> ()
                n180 = local write "三点标液2"(w328) -> ()
              }
            }
            n181 = call "Add State to Queue.vi"("State(s) In (\"\")"=w315) -> ("States Out"=w316:string)  [unwired: 14 in]
          }
          event "三点标液3": Value Change {
            n182 = event-data() -> ("NewVal"=w332:u16)  [unwired: 1 in, 5 out]
            n183 = case shown="3..7" w332 {
              frame 0, 1, Default {
                w333 = u16 2 items=["TECH4.00", "TECH7.00", "TECH10.00", "NIST1.68", "NIST4.01", "NIST6.86", "NIST9.18", "NIST12.68"] ("标液2")
                w334 = u16 0 items=["TECH4.00", "TECH7.00", "TECH10.00", "NIST1.68", "NIST4.01", "NIST6.86", "NIST9.18", "NIST12.68"] ("标液3")
                w335 = u16 1 items=["TECH4.00", "TECH7.00", "TECH10.00", "NIST1.68", "NIST4.01", "NIST6.86", "NIST9.18", "NIST12.68"] ("标液2")
                n184 = local write "三点标液3"(w334) -> ()
                n185 = local write "三点标液2"(w335) -> ()
                n186 = local write "三点标液1"(w333) -> ()
              }
              frame 2 {
                w336 = u16 0 items=["TECH4.00", "TECH7.00", "TECH10.00", "NIST1.68", "NIST4.01", "NIST6.86", "NIST9.18", "NIST12.68"] ("标液2")
                w337 = u16 2 items=["TECH4.00", "TECH7.00", "TECH10.00", "NIST1.68", "NIST4.01", "NIST6.86", "NIST9.18", "NIST12.68"] ("标液3")
                w338 = u16 1 items=["TECH4.00", "TECH7.00", "TECH10.00", "NIST1.68", "NIST4.01", "NIST6.86", "NIST9.18", "NIST12.68"] ("标液2")
                n187 = local write "三点标液3"(w337) -> ()
                n188 = local write "三点标液2"(w338) -> ()
                n189 = local write "三点标液1"(w336) -> ()
              }
              frame 3..7 {
                n190 = local read "三点标液1"() -> (w341:u16)
                n191 = local read "三点标液2"() -> (w340:u16)
                n192 = Less?(x=w341, y=w340) -> (x < y?=w339:bool)
                n193 = case shown="假" w339 {
                  frame False {
                  }
                  frame True {
                    n194 = local read "三点标液3"() -> (w344:u16)
                    n195 = local read "三点标液2"() -> (w342:u16)
                    n196 = Less Or Equal?(x=w344, y=w342) -> (x <= y?=w343:bool)
                    n197 = case shown="真" w343 {
                      tunnel: w342 -> [_ w346]
                      frame False {
                      }
                      frame True {
                        n198 = Increment(x=w346) -> (x+1=w345:u16)
                        n199 = local write "三点标液3"(w345) -> ()
                      }
                    }
                  }
                }
              }
            }
            n200 = call "Add State to Queue.vi"("State(s) In (\"\")"=w329) -> ("States Out"=w330:string)  [unwired: 14 in]
          }
          event "标液1", "标液2", "偏移值补偿": Mouse Down {
            n201 = event-data() -> ("CtlRef"=w351:refnum<vi>)  [unwired: 1 in, 7 out]
            n202 = property on="校准模式" class="Enum (严格)"() -> ("DisabledEnum"=w349:T3)  [unwired: 2 in, 2 out]
            n203 = case shown="\"Enabled\"" w349 {
              tunnel: w351 -> [w355 _]
              frame "Enabled" {
                n204 = property class="DigNum (严格)"(reference=w355) -> (reference out=w352:refnum<vi>, "Value"=w353:dbl)  [unwired: 1 in, 1 out]
                n205 = call "数字键盘.vi"("OldNumber"=w353) -> ("NewNumber"=w354:dbl)  [unwired: 1 in]
                n206 = property class="DigNum (严格)"(reference=w352, "Val(Sgnl)"=w354) -> ()  [unwired: 1 in, 2 out]
              }
              frame "Disabled", Default {
              }
            }
            n207 = call "Add State to Queue.vi"("State(s) In (\"\")"=w347) -> ("States Out"=w348:string)  [unwired: 14 in]
          }
          event "偏移值补偿": Value Change {
            n208 = event-data() -> ("NewVal"=w357:dbl)  [unwired: 1 in, 5 out]
            n209 = global read "多参数全局变量.vi" "MB session in"() -> (w358:refnum<class "MB_Master.lvclass">)
            n210 = call "000CH_pH_pH偏移修正值写入.vi"("数值"=w357, "MB session in"=w358) -> ("error out"=w356:errorcluster)  [unwired: 8 in, 1 out]
            n211 = call "Add State to Queue.vi"("State(s) In (\"\")"=w361) -> ("States Out"=w360:string)  [unwired: 14 in]
          }
          event "标液1": Value Change {
            n212 = event-data() -> ("NewVal"=w367:dbl)  [unwired: 1 in, 5 out]
            n213 = global read "多参数全局变量.vi" "MB session in"() -> (w365:refnum<class "MB_Master.lvclass">)
            n214 = call "0030H_pH_第一点标准值写入.vi"("数值"=w367, "MB session in"=w365) -> ("error out"=w366:errorcluster)  [unwired: 8 in, 1 out]
            n215 = call "Add State to Queue.vi"("State(s) In (\"\")"=w362) -> ("States Out"=w363:string)  [unwired: 14 in]
          }
          event "标液2": Value Change {
            n216 = event-data() -> ("NewVal"=w373:dbl)  [unwired: 1 in, 5 out]
            n217 = global read "多参数全局变量.vi" "MB session in"() -> (w371:refnum<class "MB_Master.lvclass">)
            n218 = call "Add State to Queue.vi"("State(s) In (\"\")"=w368) -> ("States Out"=w369:string)  [unwired: 14 in]
            n219 = call "0033H_pH_第二点标准值写入.vi"("数值"=w373, "MB session in"=w371) -> ("error out"=w372:errorcluster)  [unwired: 8 in, 1 out]
          }
          event "刷新按钮": Value Change {
            n220 = event-data() -> ()  [unwired: 1 in, 6 out]
            n221 = call "Add State to Queue.vi"("State(s) In (\"\")"=w376) -> ("States Out"=w375:string)  [unwired: 14 in]
            n222 = Two Button Dialog(message="请再次确实是否恢复出厂设置！" ("消息")) -> (T button?=w378:bool)  [unwired: 2 in]
            n223 = case shown="真" w378 {
              frame False {
              }
              frame True {
                w379 = u16 33 items=["Factory Reset"=33] ("数值")
                n224 = global read "多参数全局变量.vi" "MB session in"() -> (w380:refnum<class "MB_Master.lvclass">)
                n225 = call "0026H_pH_命令寄存器写入.vi"("数值"=w379, "MB session in"=w380) -> ()  [unwired: 8 in, 2 out]
              }
            }
          }
          event "校准启动": Value Change {
            n226 = event-data() -> ()  [unwired: 1 in, 6 out]
            n227 = global read "多参数全局变量.vi" "校准运行状态"() -> (w382:T4)
            n228 = Bundle By Name(cluster=w382, "ph"=TRUE) -> (w383:T4)
            n229 = call "Add State to Queue.vi"("State(s) In (\"\")"=w387, "State(s) At Back (\"\")"="init: all\nCal: Place standard solution\n Cal: Calibration process\nidle" ("State(s) In (\"\")")) -> ("States Out"=w386:string)  [unwired: 13 in]
            n230 = global write "多参数全局变量.vi" "校准运行状态"(w383) -> ()
          }
          event "校准停止": Value Change {
            n231 = event-data() -> ()  [unwired: 1 in, 6 out]
            n232 = call "Add State to Queue.vi"("State(s) In (\"\")"="init: all\nCal: Over\nidle" ("State(s) In (\"\")")) -> ("States Out"=w389:string)  [unwired: 14 in]
          }
        }
      }
    }
  }
  n233 = while {
    stop <- FALSE stop-if-true
    n234 = global read "多参数全局变量.vi" "权限"() -> (w394:enum16{"一级权限", "二级权限", "三级权限"})
    n235 = Wait (ms)(milliseconds to wait=u32 1000 ("等待时间（毫秒）")) -> ()  [unwired: 1 out]
    n236 = Not Equal?(x=w394, y=enum16{"一级权限", "二级权限", "三级权限"}."一级权限") -> (x != y?=w392:bool)
    n237 = property on="偏移值补偿" class="DigNum (严格)"("Visible"=w392) -> ()  [unwired: 2 in, 2 out]
  }
